vi "Create Log File Path.vi"(8 "error in":errorcluster) -> (0 "error out":errorcluster, 3 "logger path":path)   [LabVIEW 2021, in "Event Logger.lvlib"]
uses:
  Event Logger.lvlib
  <vilib>/Utility/sysdir.llb/System Directory Type.ctl
  Converter/Path Functions/Path Functions.lvlib
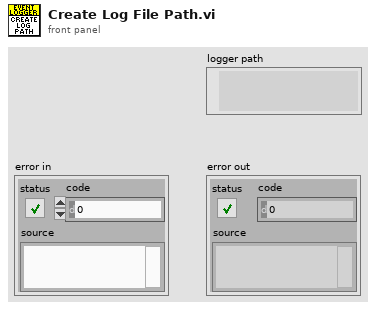
[diagram p1: front panel]
types:
  T1 = typedef "System Directory Type.ctl" = i32
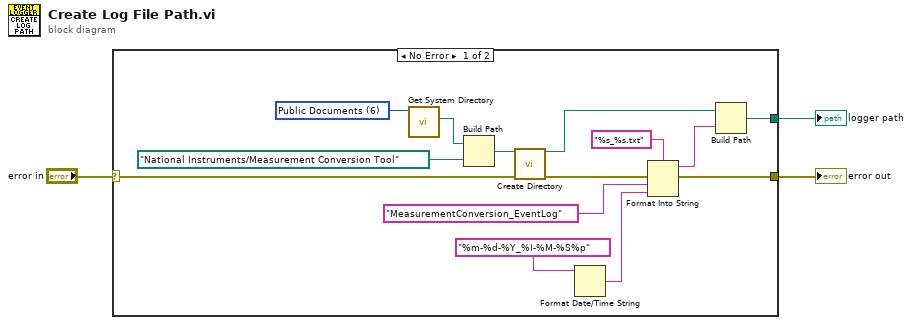
[diagram p0: block diagram]
diagram:
  n1 = case shown="No Error" "error in" {
    selector: "error in" -> [w10 w18]
    tunnel: [w17 _] -> w2
    tunnel: [w12 w18] -> w1
    frame No Error {
      w7 = T1 6 items=["User Home"=0, "User Desktop"=1, "User Documents"=2, "User Application Data"=3, "User Preferences"=4, "User Temporary"=5, "Public Documents"=6, "Public Application Data"=7, "Public Preferences"=8, "Public Cache"=13, "System Core Libraries"=9, "System Installed Libraries"=10, "Application Files"=11, "Boot Volume Root"=12] ("system directory type")
      n2 = call <vilib>:"Get System Directory.vi"("system directory type"=w7) -> ("system directory"=w9:path)  [unwired: 10 in]
      n3 = Build Path(base path=w9, name or relative path=path "National Instruments/Measurement Conversion Tool" ("Application Directory")) -> (appended path=w6:path)
      n4 = call "Create Directory.vi"("directory"=w6, "error in"=w10) -> ("dup directory"=w13:path, "error out"=w11:errorcluster)  [unwired: 12 in]
      n5 = Format Date/Time String(time format string (%c)="%m-%d-%Y_%I-%M-%S%p") -> (date/time string=w14:string)  [unwired: 2 in]
      n6 = Format Into String(format string="%s_%s.txt", error in=w11, "MeasurementConversion_EventLog" ("name"), w14) -> (resulting string=w4:string, error out=w12:errorcluster)  [unwired: 1 in]
      n7 = Build Path(base path=w13, name or relative path=w4) -> (appended path=w17:path)
    }
    frame Error {
    }
  }
  "logger path" <- w2
  "error out" <- w1
